vi "FrameReader.vi"(0 "Brightness::Value":i64=133 min=30 max=255 step=1, 1 "Contrast::Value":dbl=0.05 min=0.0 max=0.1, 2 "Exposure::Mode":u32(ring)=2 items=["Auto"=1, "Manual"=2], 3 "Exposure::Value":dbl=0.00048828125 min=0.00048828125 max=2.0, 4 "Saturation::Value":i64=83 min=0 max=200 step=1, 5 "Stop (F)":bool, 6 "Sharpness::Value":i64=25 min=0 max=50 step=1, 7 "error in":errorcluster, 8 "White Balance::Mode":u32(ring)=2 items=["Auto"=1, "Manual"=2], 9 "White Balance::Value":i64=3040 min=2800 max=10000 step=1, 10 "Interface Name":string="cam0", 11 "OK Button":bool) -> (20 "Image Out":T1(plugin-control), 21 "All Image Buffers Out":T1[](array[typedef]), 22 "Image Number":u32, 23 "Lost Image Count":u32, 24 "Total Images Transferred":u32, 25 "Frame Rate":dbl, 26 "Stopped":bool, 27 "error out":errorcluster)   [LabVIEW 2014]
doc: "Creates, and edits acquisitions using the NI Vision Acquisition Express VI.\n\nThe NI Vision Acquisition Wizard is launched by placing the Express VI on the block diagram. Select an acquisition source and configure an acquisition using NI-IMAQ, NI-IMAQdx, or simulate an acquisition by reading an AVI or image files from a folder. After an acquisition is configured, select controls and indicators to be able to programmatically set in LabVIEW. Double-click the Vision Acquisition Express VI to edit the acquisition.\n\nNote: Any images created by the Express VI need to be disposed after use. Use the IMAQ Dispose.vi to cleanup the images output by the Express VI when they are no longer needed."
uses:
  <vilib>/vision/Image Controls.llb/IMAQ Image.ctl
  <vilib>/vision/driver/IMAQdx.llb/IMAQdx Buffer Number Mode.ctl
  <vilib>/vision/driver/NI_Vision_Acquisition_Software.lvlib
  <resource>/objmgr/imaqdx.rc
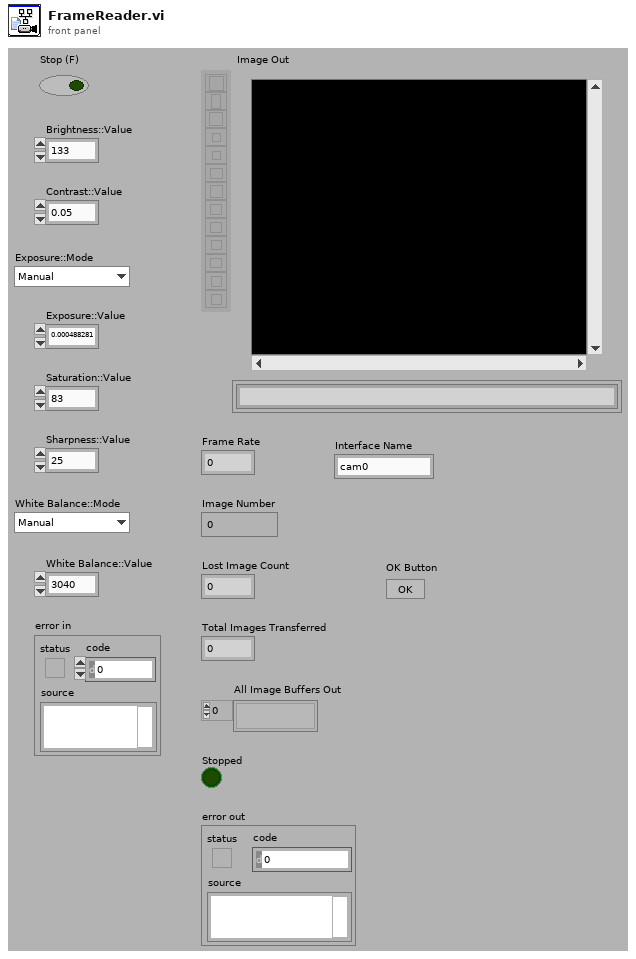
[diagram p1: front panel]
types:
  T1 = typedef "IMAQ Image.ctl" = refnum<image>
  T2 = typedef "NI_Vision_Acquisition_Software.lvlib/IMAQdx Buffer Number Mode.ctl" = enum32{"Next", "Last", "Buffer Number"}
  T3 = typedef "IMAQdx.ctl" = refnum<k21>
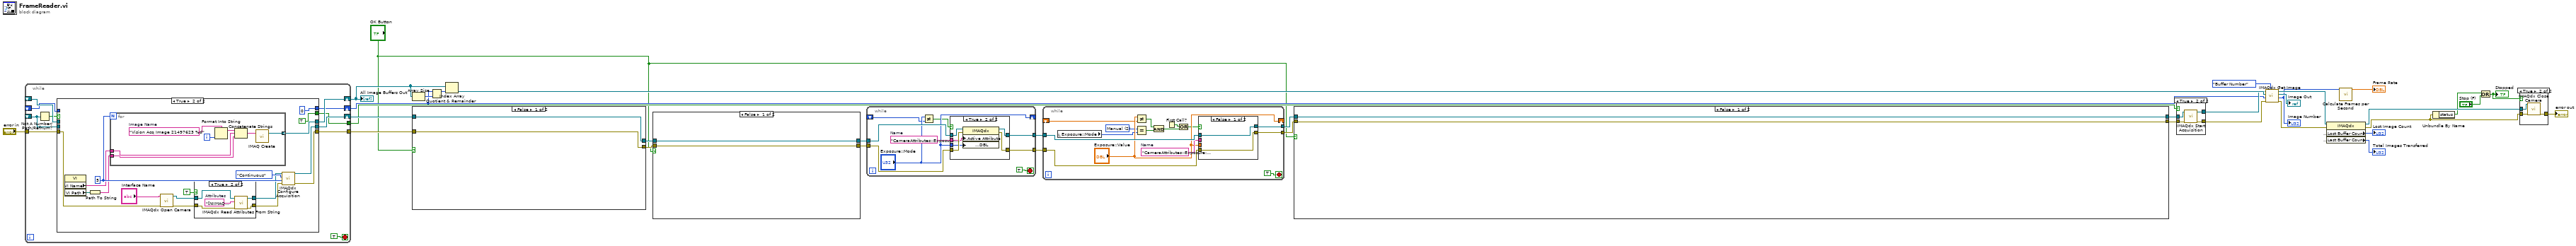
[diagram p0: block diagram]
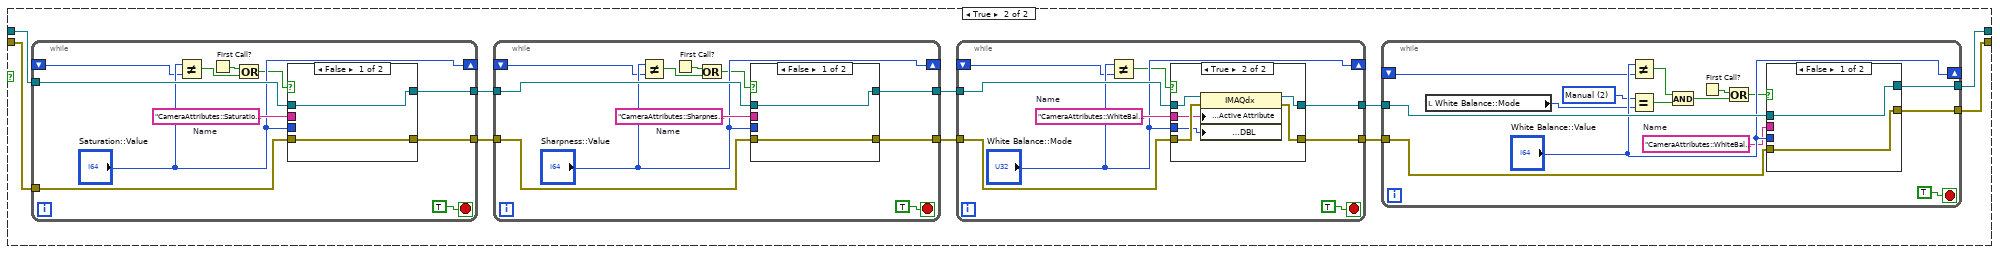
[diagram p2: hidden frame]
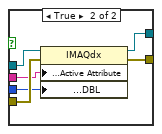
[diagram p3: hidden frame]
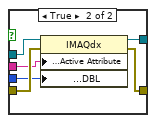
[diagram p5: hidden frame]
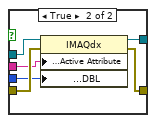
[diagram p6: hidden frame]
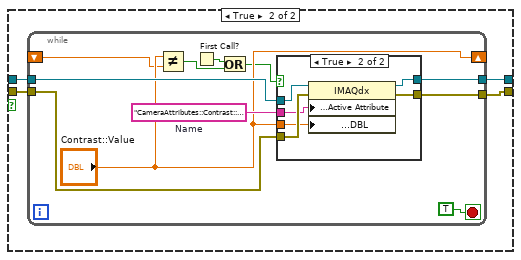
[diagram p7: hidden frame]
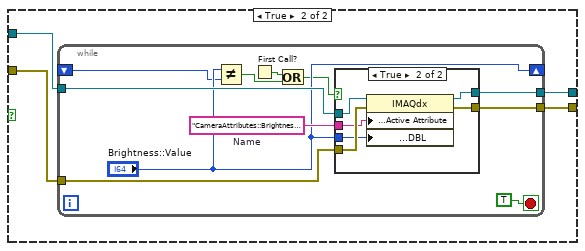
[diagram p9: hidden frame]
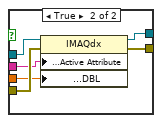
[diagram p13: hidden frame]
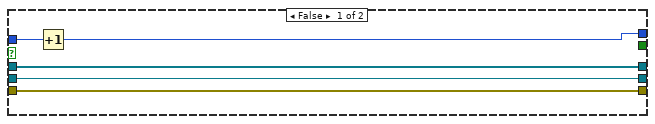
[diagram p15: hidden frame]
diagram:
  n1 = while {
    shift-right: [w47] -> w34
    shift-left: _ -> [w39]
    tunnel: [w46] -> w35
    tunnel: "error in" -> [w45]
    shift-right: [w43] -> w18
    shift-left: _ -> [w42]
    shift-right: [w41] -> w11
    shift-left: _ -> [w40]
    tunnel: [w37] -> w10
    stop <- TRUE stop-if-true
    n2 = Not A Number/Path/Refnum?(number/path/refnum=w39) -> (NaN/Path/Refnum?=w38:bool)
    n3 = case shown="True" w38 {
      tunnel: [w52 w67] -> w47
      tunnel: w39 -> [w52 _]
      tunnel: [w51 w66] -> w46
      tunnel: w45 -> [w51 w69]
      tunnel: [w50 w65] -> w43
      tunnel: w42 -> [w50 _]
      tunnel: [w48 0] -> w41
      tunnel: w40 -> [w49 _]
      tunnel: [_ TRUE] -> w37
      frame False {
        n4 = Increment(x=w49) -> (x+1=w48:i32)
      }
      frame True {
        w64 = u32 5 ("Number of Image Buffers")
        n5 = property class="VI"() -> ("VI Name"=w60:string, "VI Path"=w61:path)  [unwired: 2 in, 2 out]
        n6 = Path To String(path=w61) -> (string=w59:string)
        n7 = for "For Loop_template0" {
          N: w64 -> [_]
          tunnel: [w83] -> w65 mode=indexing
          tunnel: w60 -> [w78]
          tunnel: w59 -> [w77]
          i -> [w82]
          w81 = "Vision Acq Image 21497623 %d"  # Image Name
          n8 = Format Into String(format string=w81, w82) -> (resulting string=w80:string)  [unwired: 2 in, 1 out]
          n9 = Concatenate Strings(w80, w78, w77) -> (w79:string)
          n10 = call "IMAQ Create"("Image Name"=w79) -> ("New Image"=w83:T1)  [unwired: 3 in, 2 out]
        }
        n11 = call <vilib>:"IMAQdx Open Camera.vi"("error in"=w69, "Session In"="Interface Name") -> ("error out"=w57:errorcluster, "Session Out"=w58:T3)  [unwired: 1 in, 7 out]
        n12 = case shown="True" TRUE ("Init Attributes") {
          tunnel: w58 -> [w71 w76]
          tunnel: w57 -> [w70 w75]
          tunnel: [w71 w73] -> w56
          tunnel: [w70 w72] -> w55
          frame False {
          }
          frame True {
            w74 = "[NIIMAQ_HEADER]\nType = 2\nVersion = 8\n\n[CAMERA_DATA]\nAcquisitionAttributes::Bayer::Algorithm = \"Bilinear\"\nAcquisitionAttributes::Bayer::GainB = \"1\"\nAcquisitionAttributes::Bayer::GainG = \"1\"\nAcquisitionAttributes::Bayer::GainR = \"1\"\nAcquisitionAttributes::Bayer::Pattern = \"Use hardware value\"\nAcquisitionAttributes::BitsPerPixel = \"Use hardware value\"\nAcquisitionAttributes::IgnoreFirstFrame = \"false\"\nAcquisitionAttributes::ImageDecoderCopyMode = \"Auto\"\nAcquisitionAttributes::OutputImageType = \"Auto\"\nAcquisitionAttributes::OverwriteMode = \"Get Newest\"\nAcquisitionAttributes::PixelSignedness = \"Signed\"\nAcquisitionAttributes::ReceiveTimestampMode = \"None\"\nAcquisitionAttributes::ShiftPixelBits = \"false\"\nAcquisitionAttributes::SwapPixelBytes = \"false\"\nAcquisitionAttributes::Timeout = \"5000\"\nAcquisitionAttributes::VerticalMirror = \"false\"\nAcquisitionAttributes::VideoMode = \"1280x720 RGB24 30.00fps\"\nCameraAttributes::BacklightCompensation::Mode = \"Manual\"\nCameraAttributes::BacklightCompensation::Value = \"false\"\nCameraAttributes::Brightness::Mode = \"Manual\"\nCameraAttributes::Brightness::Value = \"133\"\nCameraAttributes::Contrast::Mode = \"Manual\"\nCameraAttributes::Contrast::Value = \"0.050000000000000003\"\nCameraAttributes::Exposure::Mode = \"Manual\"\nCameraAttributes::Exposure::Value = \"0.00048828125\"\nCameraAttributes::Pan::Mode = \"Manual\"\nCameraAttributes::Pan::Value = \"0\"\nCameraAttributes::Saturation::Mode = \"Manual\"\nCameraAttributes::Saturation::Value = \"83\"\nCameraAttributes::Sharpness::Mode = \"Manual\"\nCameraAttributes::Sharpness::Value = \"25\"\nCameraAttributes::Tilt::Mode = \"Manual\"\nCameraAttributes::Tilt::Value = \"0\"\nCameraAttributes::WhiteBalance::Mode = \"Manual\"\nCameraAttributes::WhiteBalance::Value = \"3040\"\nCameraAttributes::Zoom::Mode = \"Manual\"\nCameraAttributes::Zoom::Value = \"0\"\n"  # Attributes
            n13 = call <vilib>:"IMAQdx Read Attributes From String.vi"("error in"=w75, "Attributes String In"=w74, "Session In"=w76) -> ("error out"=w72:errorcluster, "Session Out"=w73:T3)  [unwired: 7 out]
          }
        }
        n14 = call <vilib>:"IMAQdx Configure Acquisition.vi"("error in"=w55, "Number of Buffers"=w64, "Continuous?"=enum32{"One Shot", "Continuous"}."Continuous" ("Mode"), "Session In"=w56) -> ("error out"=w66:errorcluster, "Session Out"=w67:T3)  [unwired: 6 out]
      }
    }
  }
  "All Image Buffers Out" <- w18
  n15 = Array Size(array=w18) -> (size(s)=w19:i32)
  n16 = case shown="False" "OK Button" {
    tunnel: w35 -> [w84 w89]
    tunnel: w34 -> [w85 w88]
    tunnel: [w84 w87] -> w33
    tunnel: [w85 w86] -> w32
    frame False {
    }
    frame True {
      n17 = while {
        tunnel: w89 -> [w100]
        tunnel: [w99] -> w86
        tunnel: w88 -> [w98]
        tunnel: [w97] -> w87
        shift-right: ["Brightness::Value"] -> _
        shift-left: _ -> [w93]
        stop <- TRUE stop-if-true
        w96 = "CameraAttributes::Brightness::Value"  # Name
        n18 = Not Equal?(x="Brightness::Value", y=w93) -> (x != y?=w92:bool)
        n19 = First Call?() -> (First Call?: T/F=w91:bool)
        n20 = Or(x=w91, y=w92) -> (x .or. y?=w90:bool)
        n21 = case shown="True" w90 {
          tunnel: w100 -> [w101 w108]
          tunnel: [w102 w107] -> w99
          tunnel: w98 -> [w102 w106]
          tunnel: [w101 w105] -> w97
          tunnel: w96 -> [_ w104]
          tunnel: "Brightness::Value" -> [_ w103]
          frame False {
          }
          frame True {
            n22 = property class="IMAQdx"(reference=w106, error in=w108, "Camera Attributes:Active Attribute"=w104, "Camera Attributes:Value:DBL"=w103) -> (reference out=w107:T3, error out=w105:errorcluster)
          }
        }
      }
    }
  }
  n23 = Quotient & Remainder(x=w11, y=w19) -> (x-y*floor(x/y)=w17:i32)  [unwired: 1 out]
  n24 = Index Array(array=w18, index=w17) -> (element=w16:T1)
  n25 = case shown="False" "OK Button" {
    tunnel: w33 -> [w109 w114]
    tunnel: w32 -> [w110 w113]
    tunnel: [w109 w112] -> w31
    tunnel: [w110 w111] -> w30
    frame False {
    }
    frame True {
      n26 = while {
        tunnel: w114 -> [w125]
        tunnel: [w124] -> w111
        tunnel: w113 -> [w123]
        tunnel: [w122] -> w112
        shift-right: ["Contrast::Value"] -> _
        shift-left: _ -> [w118]
        stop <- TRUE stop-if-true
        w121 = "CameraAttributes::Contrast::Value"  # Name
        n27 = Not Equal?(x="Contrast::Value", y=w118) -> (x != y?=w116:bool)
        n28 = First Call?() -> (First Call?: T/F=w117:bool)
        n29 = Or(x=w117, y=w116) -> (x .or. y?=w115:bool)
        n30 = case shown="True" w115 {
          tunnel: w125 -> [w126 w133]
          tunnel: [w127 w132] -> w124
          tunnel: w123 -> [w127 w131]
          tunnel: [w126 w130] -> w122
          tunnel: w121 -> [_ w129]
          tunnel: "Contrast::Value" -> [_ w128]
          frame False {
          }
          frame True {
            n31 = property class="IMAQdx"(reference=w131, error in=w133, "Camera Attributes:Active Attribute"=w129, "Camera Attributes:Value:DBL"=w128) -> (reference out=w132:T3, error out=w130:errorcluster)
          }
        }
      }
    }
  }
  n32 = while {
    tunnel: w31 -> [w142]
    tunnel: [w141] -> w28
    tunnel: w30 -> [w140]
    tunnel: [w139] -> w29
    shift-right: ["Exposure::Mode"] -> _
    shift-left: _ -> [w135]
    stop <- TRUE stop-if-true
    w138 = "CameraAttributes::Exposure::Mode"  # Name
    n33 = Not Equal?(x="Exposure::Mode", y=w135) -> (x != y?=w134:bool)
    n34 = case shown="True" w134 {
      tunnel: w142 -> [w143 w150]
      tunnel: [w144 w149] -> w141
      tunnel: w140 -> [w144 w148]
      tunnel: [w143 w147] -> w139
      tunnel: w138 -> [_ w146]
      tunnel: "Exposure::Mode" -> [_ w145]
      frame False {
      }
      frame True {
        n35 = property class="IMAQdx"(reference=w148, error in=w150, "Camera Attributes:Active Attribute"=w146, "Camera Attributes:Value:DBL"=w145) -> (reference out=w149:T3, error out=w147:errorcluster)
      }
    }
  }
  n36 = while {
    tunnel: w29 -> [w165]
    tunnel: [w164] -> w26
    tunnel: w28 -> [w163]
    tunnel: [w162] -> w27
    shift-right: ["Exposure::Value"] -> _
    shift-left: _ -> [w158]
    stop <- TRUE stop-if-true
    w155 = u32 2 items=["Auto"=1, "Manual"=2] ("Exposure::Mode")
    w161 = "CameraAttributes::Exposure::Value"  # Name
    n37 = local read "Exposure::Mode"() -> (w156:u32)
    n38 = Not Equal?(x="Exposure::Value", y=w158) -> (x != y?=w154:bool)
    n39 = Equal?(x=w155, y=w156) -> (x = y?=w153:bool)
    n40 = And(x=w154, y=w153) -> (x .and. y?=w152:bool)
    n41 = First Call?() -> (First Call?: T/F=w157:bool)
    n42 = Or(x=w157, y=w152) -> (x .or. y?=w151:bool)
    n43 = case shown="False" w151 {
      tunnel: w165 -> [w166 w173]
      tunnel: [w167 w172] -> w164
      tunnel: w163 -> [w167 w171]
      tunnel: [w166 w170] -> w162
      tunnel: w161 -> [_ w169]
      tunnel: "Exposure::Value" -> [_ w168]
      frame False {
      }
      frame True {
        n44 = property class="IMAQdx"(reference=w171, error in=w173, "Camera Attributes:Active Attribute"=w169, "Camera Attributes:Value:DBL"=w168) -> (reference out=w172:T3, error out=w170:errorcluster)
      }
    }
  }
  n45 = case shown="False" "OK Button" {
    tunnel: w27 -> [w174 w185]
    tunnel: w26 -> [w175 w184]
    tunnel: [w174 w177] -> w25
    tunnel: [w175 w176] -> w14
    frame False {
    }
    frame True {
      n46 = while {
        tunnel: w185 -> [w255]
        tunnel: [w254] -> w182
        tunnel: w184 -> [w253]
        tunnel: [w252] -> w183
        shift-right: ["Saturation::Value"] -> _
        shift-left: _ -> [w248]
        stop <- TRUE stop-if-true
        w251 = "CameraAttributes::Saturation::Value"  # Name
        n47 = Not Equal?(x="Saturation::Value", y=w248) -> (x != y?=w246:bool)
        n48 = First Call?() -> (First Call?: T/F=w247:bool)
        n49 = Or(x=w247, y=w246) -> (x .or. y?=w245:bool)
        n50 = case shown="False" w245 {
          tunnel: w255 -> [w256 w263]
          tunnel: [w257 w262] -> w254
          tunnel: w253 -> [w257 w261]
          tunnel: [w256 w260] -> w252
          tunnel: w251 -> [_ w259]
          tunnel: "Saturation::Value" -> [_ w258]
          frame False {
          }
          frame True {
            n51 = property class="IMAQdx"(reference=w261, error in=w263, "Camera Attributes:Active Attribute"=w259, "Camera Attributes:Value:DBL"=w258) -> (reference out=w262:T3, error out=w260:errorcluster)
          }
        }
      }
      n52 = while {
        tunnel: w183 -> [w236]
        tunnel: [w235] -> w180
        tunnel: w182 -> [w234]
        tunnel: [w233] -> w181
        shift-right: ["Sharpness::Value"] -> _
        shift-left: _ -> [w229]
        stop <- TRUE stop-if-true
        w232 = "CameraAttributes::Sharpness::Value"  # Name
        n53 = Not Equal?(x="Sharpness::Value", y=w229) -> (x != y?=w227:bool)
        n54 = First Call?() -> (First Call?: T/F=w228:bool)
        n55 = Or(x=w228, y=w227) -> (x .or. y?=w226:bool)
        n56 = case shown="False" w226 {
          tunnel: w236 -> [w237 w244]
          tunnel: [w238 w243] -> w235
          tunnel: w234 -> [w238 w242]
          tunnel: [w237 w241] -> w233
          tunnel: w232 -> [_ w240]
          tunnel: "Sharpness::Value" -> [_ w239]
          frame False {
          }
          frame True {
            n57 = property class="IMAQdx"(reference=w242, error in=w244, "Camera Attributes:Active Attribute"=w240, "Camera Attributes:Value:DBL"=w239) -> (reference out=w243:T3, error out=w241:errorcluster)
          }
        }
      }
      n58 = while {
        tunnel: w181 -> [w217]
        tunnel: [w216] -> w178
        tunnel: w180 -> [w215]
        tunnel: [w214] -> w179
        shift-right: ["White Balance::Mode"] -> _
        shift-left: _ -> [w210]
        stop <- TRUE stop-if-true
        w213 = "CameraAttributes::WhiteBalance::Mode"  # Name
        n59 = Not Equal?(x="White Balance::Mode", y=w210) -> (x != y?=w209:bool)
        n60 = case shown="True" w209 {
          tunnel: w217 -> [w218 w225]
          tunnel: [w219 w224] -> w216
          tunnel: w215 -> [w219 w223]
          tunnel: [w218 w222] -> w214
          tunnel: w213 -> [_ w221]
          tunnel: "White Balance::Mode" -> [_ w220]
          frame False {
          }
          frame True {
            n61 = property class="IMAQdx"(reference=w223, error in=w225, "Camera Attributes:Active Attribute"=w221, "Camera Attributes:Value:DBL"=w220) -> (reference out=w224:T3, error out=w222:errorcluster)
          }
        }
      }
      n62 = while {
        tunnel: w179 -> [w200]
        tunnel: [w199] -> w176
        tunnel: w178 -> [w198]
        tunnel: [w197] -> w177
        shift-right: ["White Balance::Value"] -> _
        shift-left: _ -> [w194]
        stop <- TRUE stop-if-true
        w191 = u32 2 items=["Auto"=1, "Manual"=2] ("Exposure::Mode")
        w193 = "CameraAttributes::WhiteBalance::Value"  # Name
        n63 = local read "White Balance::Mode"() -> (w190:u32)
        n64 = Not Equal?(x="White Balance::Value", y=w194) -> (x != y?=w188:bool)
        n65 = Equal?(x=w191, y=w190) -> (x = y?=w189:bool)
        n66 = And(x=w188, y=w189) -> (x .and. y?=w187:bool)
        n67 = First Call?() -> (First Call?: T/F=w192:bool)
        n68 = Or(x=w192, y=w187) -> (x .or. y?=w186:bool)
        n69 = case shown="False" w186 {
          tunnel: w200 -> [w201 w208]
          tunnel: [w202 w207] -> w199
          tunnel: w198 -> [w202 w206]
          tunnel: [w201 w205] -> w197
          tunnel: w193 -> [_ w204]
          tunnel: "White Balance::Value" -> [_ w203]
          frame False {
          }
          frame True {
            n70 = property class="IMAQdx"(reference=w206, error in=w208, "Camera Attributes:Active Attribute"=w204, "Camera Attributes:Value:DBL"=w203) -> (reference out=w207:T3, error out=w205:errorcluster)
          }
        }
      }
    }
  }
  n71 = case shown="True" w10 {
    tunnel: w14 -> [w265 w269]
    tunnel: w25 -> [w264 w268]
    tunnel: [w264 w267] -> w12
    tunnel: [w265 w266] -> w13
    frame False {
    }
    frame True {
      n72 = call <vilib>:"IMAQdx Start Acquisition.vi"("error in"=w268, "Session In"=w269) -> ("error out"=w267:errorcluster, "Session Out"=w266:T3)  [unwired: 8 out]
    }
  }
  n73 = call <vilib>:"IMAQdx Get Image.vi"("Buffer Number Mode (Next)"=IMAQdx_Buffer_Number_Mode."Buffer Number", "error in"=w12, "Buffer Number In"=w11, "Image In"=w16, "Session In"=w13) -> ("error out"=w23:errorcluster, "Buffer Number Out"=w9:u32, "Image Out"=→"Image Out":T1, "Session Out"=w24:T3)  [unwired: 3 out]
  "Image Number" <- w9
  n74 = property class="IMAQdx"(reference=w24, error in=w23) -> (reference out=w6:T3, error out=w15:errorcluster, "Status Information:Lost Buffer Count"=→"Lost Image Count":u32, "Status Information:Last Buffer Count"=→"Total Images Transferred":u32)
  n75 = call <vilib>:"Calculate Frames per Second.vi"("Buffer Number"=w9) -> ("Acquired Frames/s"=→"Frame Rate":dbl)  [unwired: 2 in, 8 out]
  n76 = Unbundle By Name(w15) -> ("status"=w2:bool)
  n77 = Or(x=w2, y="Stop (F)") -> (x .or. y?=w3:bool)
  "Stopped" <- w3
  n78 = case "Case Structure_template1" shown="True" w3 {
    tunnel: [w270 w272] -> w5
    tunnel: w15 -> [w270 w273]
    tunnel: w6 -> [_ w271]
    frame False {
    }
    frame True {
      n79 = call <vilib>:"IMAQdx Close Camera.vi"("error in"=w273, "Session In"=w271) -> ("error out"=w272:errorcluster)  [unwired: 9 out]
    }
  }
  "error out" <- w5
